vi "Lua_Load_And_Start.vi"(3 "error in (no error)":errorcluster, 4 "Lua Script":string, 5 "Handle In":i32) -> (0 "error out":errorcluster, 1 "Debug Message":string="LUA_DEBUG_DATA", 2 "Handle Out":i32)   [LabVIEW 2020]
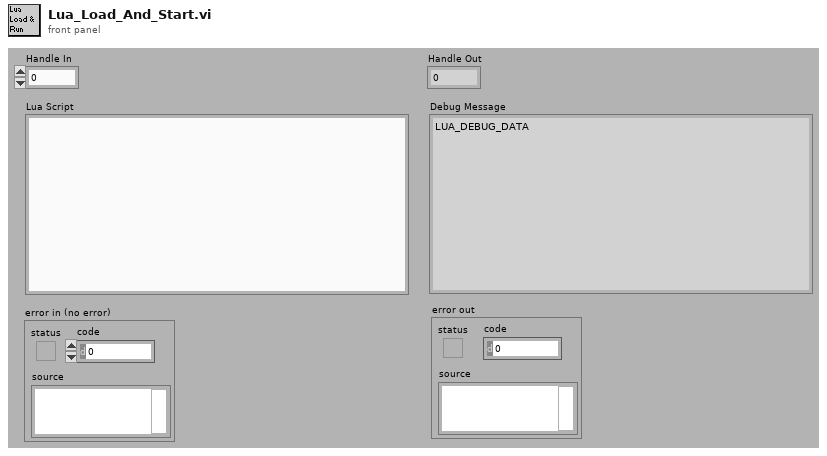
[diagram p1: front panel]
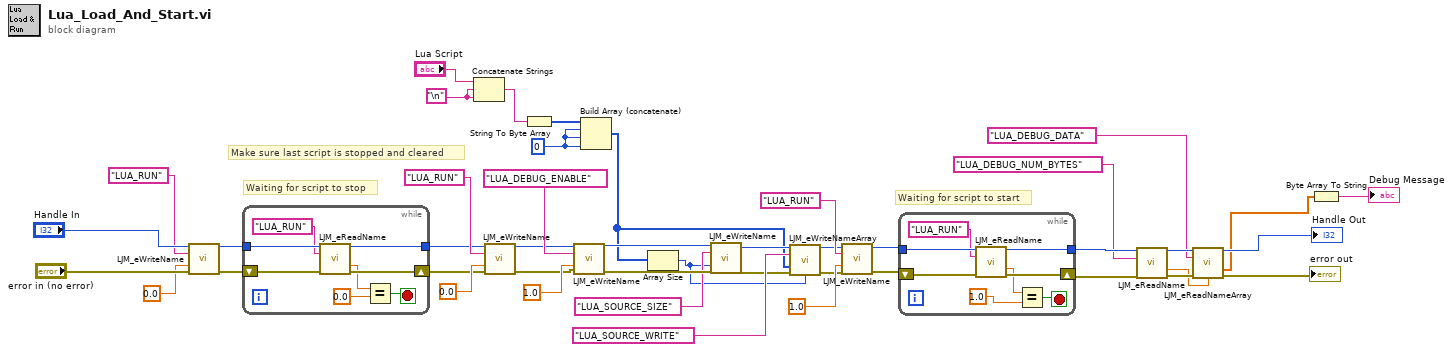
[diagram p0: block diagram]
diagram:
  w13 = "\n"
  w18 = 0
  # "Make sure last script is stopped and cleared"
  # "Waiting for script to start"
  # "Waiting for script to stop"
  n1 = call "LJM_eWriteName.vi"("Handle In"="Handle In", "Name"="LUA_RUN", "Value"=0.0, "error in"="error in (no error)") -> ("Handle Out"=w39:i32, "error out"=w41:errorcluster)  [unwired: 10 in]
  n2 = while {
    shift-right: [w51] -> w21
    shift-left: w41 -> [w52]
    tunnel: w39 -> [w50]
    tunnel: [w48] -> w22
    stop <- w47 stop-if-true
    n3 = call "LJM_eReadName.vi"("Handle In"=w50, "Name"="LUA_RUN", "error in"=w52) -> ("Handle Out"=w48:i32, "Value"=w46:dbl, "error out"=w51:errorcluster)  [unwired: 10 in]
    n4 = Equal?(x=w46, y=0.0) -> (x = y?=w47:bool)
  }
  n5 = Concatenate Strings("Lua Script", w13, w13) -> (w16:string)
  n6 = call "LJM_eWriteName.vi"("Handle In"=w22, "Name"="LUA_RUN", "Value"=0.0, "error in"=w21) -> ("Handle Out"=w19:i32, "error out"=w20:errorcluster)  [unwired: 10 in]
  n7 = String To Byte Array(string=w16) -> (unsigned byte array=w15:u8[])
  n8 = call "LJM_eWriteName.vi"("Handle In"=w19, "Name"="LUA_DEBUG_ENABLE", "Value"=1.0, "error in"=w20) -> ("Handle Out"=w34:i32, "error out"=w36:errorcluster)  [unwired: 10 in]
  n9 = Build Array (concatenate)(w15, w18, w18, w18) -> (w17:i32[])
  n10 = Array Size(array=w17) -> (size(s)=w12:i32)
  n11 = call "LJM_eWriteName.vi"("Handle In"=w34, "Name"="LUA_SOURCE_SIZE", "Value"=w12, "error in"=w36) -> ("Handle Out"=w25:i32, "error out"=w26:errorcluster)  [unwired: 10 in]
  n12 = call "LJM_eWriteNameArray.vi"("Handle In"=w25, "Name"="LUA_SOURCE_WRITE", "aValues"=w17, "error in"=w26, "NumValues"=w12) -> ("Handle Out"=w29:i32, "error out"=w28:errorcluster)  [unwired: 8 in, 1 out]
  n13 = call "LJM_eWriteName.vi"("Handle In"=w29, "Name"="LUA_RUN", "Value"=1.0, "error in"=w28) -> ("Handle Out"=w33:i32, "error out"=w32:errorcluster)  [unwired: 10 in]
  n14 = while {
    shift-right: [w59] -> w9
    shift-left: w32 -> [w60]
    tunnel: w33 -> [w58]
    tunnel: [w56] -> w11
    stop <- w55 stop-if-true
    n15 = call "LJM_eReadName.vi"("Handle In"=w58, "Name"="LUA_RUN", "error in"=w60) -> ("Handle Out"=w56:i32, "Value"=w54:dbl, "error out"=w59:errorcluster)  [unwired: 10 in]
    n16 = Equal?(x=w54, y=1.0) -> (x = y?=w55:bool)
  }
  n17 = call "LJM_eReadName.vi"("Handle In"=w11, "Name"="LUA_DEBUG_NUM_BYTES", "error in"=w9) -> ("Handle Out"=w8:i32, "Value"=w5:dbl, "error out"=w7:errorcluster)  [unwired: 10 in]
  n18 = call "LJM_eReadNameArray.vi"("Handle In"=w8, "Name"="LUA_DEBUG_DATA", "error in"=w7, "NumValues"=w5) -> ("Handle Out"=→"Handle Out":i32, "aValues"=w1:dbl[], "error out"=→"error out":errorcluster)  [unwired: 8 in, 1 out]
  n19 = Byte Array To String(unsigned byte array=w1) -> (string=→"Debug Message":string)
